vi "SampleCalibrationRemovePlate.vi"(8 "Error In":errorcluster, 11 "MotorController in":refnum<class "MotorController.lvclass">) -> (0 "Error Out":errorcluster, 3 "MotorController out":refnum<class "MotorController.lvclass">)   [LabVIEW 2019]
uses:
  MotorController.lvclass
panel:
  in  "Next":bool
  # "Sample Calibration - Remove Grid Plate"
  # "Remove the Grid Plate if done with calibration activities."
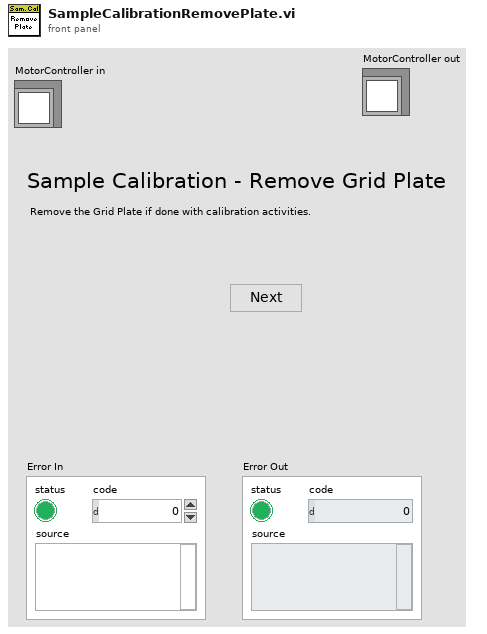
[diagram p1: front panel]
types:
  T1 = enum8{"Enabled", "Disabled", "Disabled and Grayed Out"}
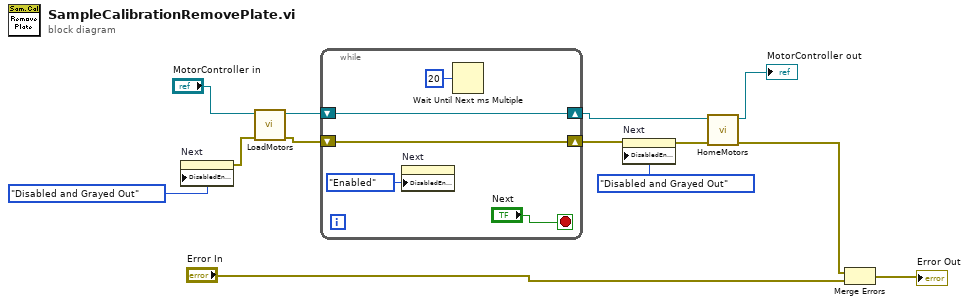
[diagram p0: block diagram]
diagram:
  n1 = property on="Next" class="Bool"("DisabledEnum"=T1."Disabled and Grayed Out" ("Disabled")) -> (error out=w1:errorcluster)  [unwired: 2 in, 1 out]
  n2 = call "LoadMotors.vi"("error in (no error)"=w1, "MotorController in"="MotorController in") -> ("error out"=w10:errorcluster, "MotorController out"=w11:refnum<class "MotorController.lvclass">)  [unwired: 8 in]
  n3 = while {
    shift-right: [w15] -> w8
    shift-left: w10 -> [w15]
    shift-right: [w16] -> w6
    shift-left: w11 -> [w16]
    stop <- "Next" stop-if-true
    n4 = property on="Next" class="Bool"("DisabledEnum"=T1."Enabled" ("Disabled")) -> ()  [unwired: 2 in, 2 out]
    n5 = Wait Until Next ms Multiple(millisecond multiple=u32 20) -> ()  [unwired: 1 out]
  }
  n6 = property on="Next" class="Bool"(error in=w8, "DisabledEnum"=T1."Disabled and Grayed Out" ("Disabled")) -> (error out=w7:errorcluster)  [unwired: 1 in, 1 out]
  n7 = call "HomeMotors.vi"("error in (no error)"=w7, "MotorController in"=w6) -> ("error out"=w3:errorcluster, "MotorController out"=→"MotorController out":refnum<class "MotorController.lvclass">)  [unwired: 8 in]
  n8 = Merge Errors(w3, "Error In") -> (→"Error Out":errorcluster)
